vi "Station - Config File.vi"(6 "Action":enum16{"Write", "Read", "Read All", "Remove"}(ring), 8 "error in (no error)":errorcluster, 9 "Value":string[](array[string]), 10 "Key Name":string[](array[string]), 11 "Station Name":string) -> (0 "error out":errorcluster, 3 "Value Out":T1(array[cluster]))   [LabVIEW 2019]
uses:
  <vilib>/Utility/config.llb/Write Key (String).vi
  <vilib>/Utility/config.llb/Read Key (String).vi
  <vilib>/Utility/config.llb/NI_LVConfig.lvlib
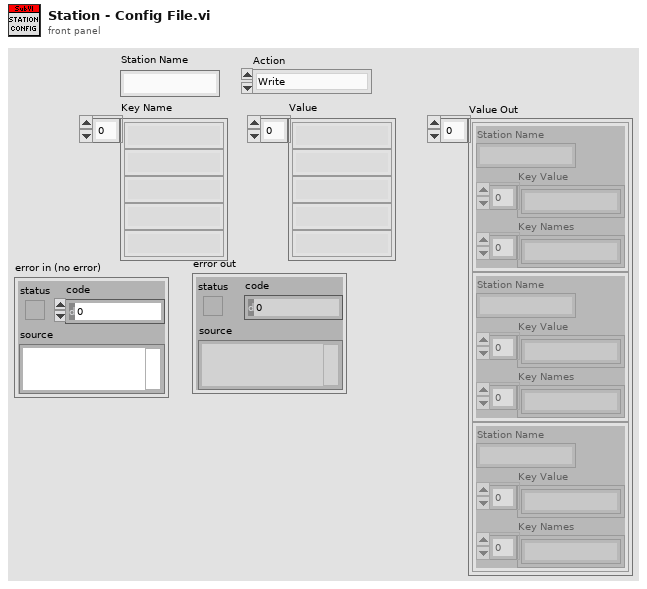
[diagram p1: front panel]
types:
  T1 = cluster{"Station Name":string, "Key Value":string[], "Key Names":string[]}[]
  T2 = typedef "NI_LVConfig.lvlib/Config Data RefNum.ctl" = refnum<k1>
  T3 = cluster{"Station Name":string, "Key Value":string[], "Key Names":string[]}
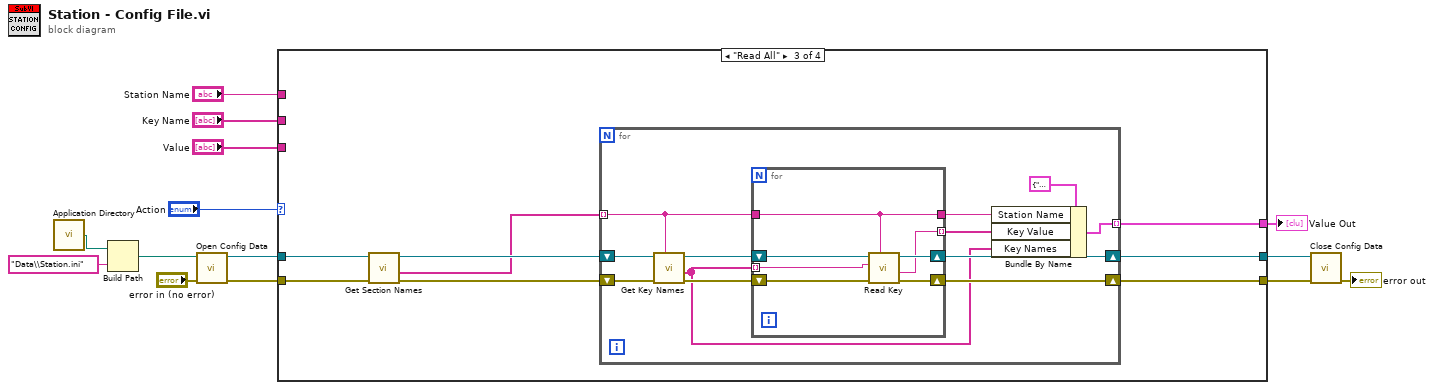
[diagram p0: block diagram]
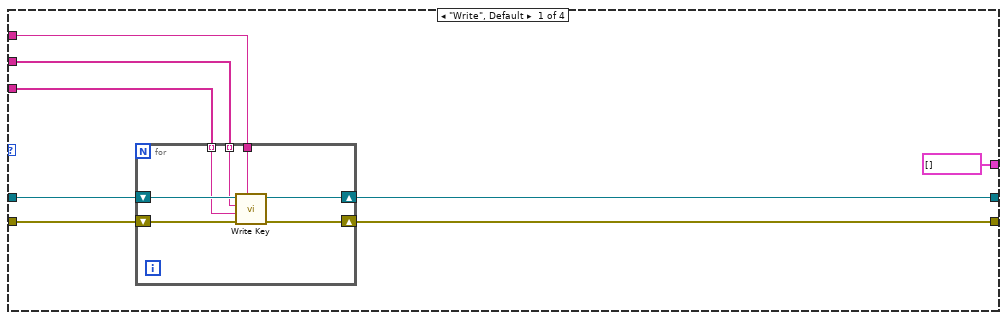
[diagram p2: hidden frame]
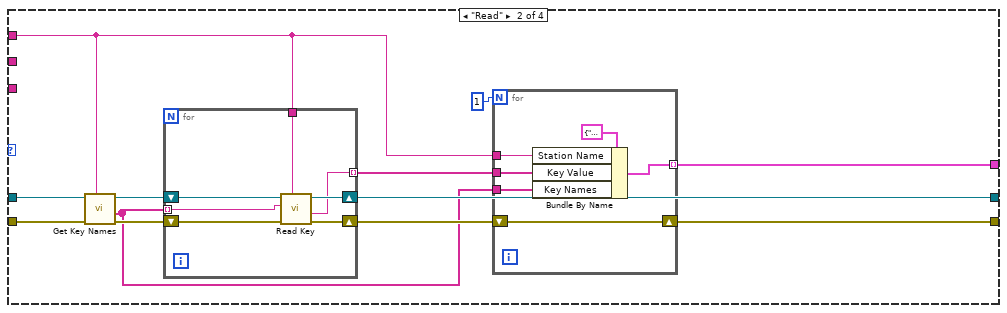
[diagram p3: hidden frame]
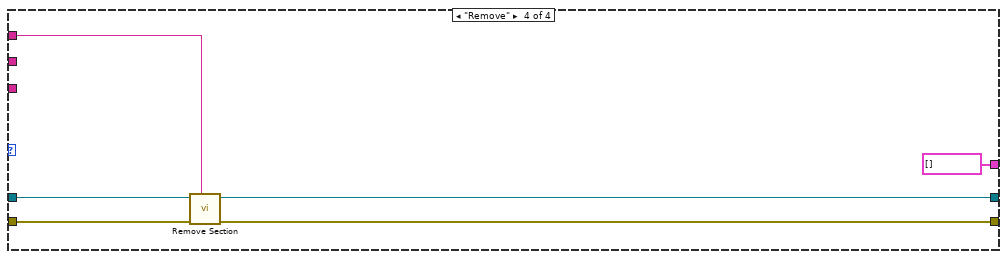
[diagram p4: hidden frame]
diagram:
  n1 = call <vilib>:"Application Directory.vi"() -> ("Application Directory"=w14:path)
  n2 = Build Path(base path=w14, name or relative path="Data\\Station.ini") -> (appended path=w1:path)
  n3 = call <vilib>:"Open Config Data.vi"("error in (no error)"="error in (no error)", "configuration file path"=w1) -> ("error out"=w12:errorcluster, "refnum"=w11:T2)  [unwired: 7 in, 1 out]
  n4 = case shown="\"Read All\"" "Action" {
    tunnel: w12 -> [w22 w34 w59 w85]
    tunnel: w11 -> [w21 w32 w58 w87]
    tunnel: [w20 w41 w61 w86] -> w10
    tunnel: [w19 w37 w62 w84] -> w9
    tunnel: "Value" -> [w18 _ _ _]
    tunnel: "Key Name" -> [w17 _ _ _]
    tunnel: "Station Name" -> [w16 w31 _ w83]
    tunnel: [T1 [] w39 w60 T1 []] -> w2
    frame "Write", Default {
      n5 = for {
        shift-right: [w26] -> w19
        shift-left: w22 -> [w29]
        shift-right: [w27] -> w20
        shift-left: w21 -> [w28]
        tunnel: w16 -> [w25]
        tunnel: w17 -> [w24] mode=indexing
        tunnel: w18 -> [w23] mode=indexing
        n6 = call-poly <vilib>:"Write Key.vi"("section"=w25, "error in (no error)"=w29, "value"=w23, "key"=w24, "refnum"=w28) -> ("error out"=w26:errorcluster, "refnum out"=w27:T2)  [unwired: 4 in, 1 out]
      }
    }
    frame "Read" {
      n7 = call <vilib>:"Get Key Names.vi"("section"=w31, "error in (no error)"=w34, "refnum"=w32) -> ("error out"=w35:errorcluster, "key names"=w30:string[], "refnum out"=w33:T2)  [unwired: 5 in, 1 out]
      n8 = for {
        tunnel: w31 -> [w50]
        shift-right: [w51] -> w41
        shift-left: w33 -> [w54]
        shift-right: [w52] -> w36
        shift-left: w35 -> [w53]
        tunnel: [w49] -> w40 mode=indexing
        tunnel: w30 -> [w48] mode=indexing
        n9 = call-poly <vilib>:"Read Key.vi"("section"=w50, "error in (no error)"=w53, "key"=w48, "refnum"=w54) -> ("error out"=w52:errorcluster, "value"=w49:string, "refnum out"=w51:T2)  [unwired: 4 in, 1 out]
      }
      n10 = for {
        N: 1 -> [_]
        tunnel: w31 -> [w47]
        tunnel: w40 -> [w46]
        tunnel: [w45] -> w39 mode=indexing
        shift-right: [w44] -> w37
        shift-left: w36 -> [w44]
        tunnel: w30 -> [w42]
        n11 = Bundle By Name(cluster=T3 {"Station Name"="", "Key Value"=[], "Key Names"=[]}, "Station Name"=w47, "Key Value"=w46, "Key Names"=w42) -> (w45:T3)
      }
    }
    frame "Read All" {
      n12 = call <vilib>:"Get Section Names.vi"("error in (no error)"=w59, "refnum"=w58) -> ("error out"=w57:errorcluster, "section names"=w55:string[], "refnum out"=w56:T2)  [unwired: 7 in]
      n13 = for {
        tunnel: [w64] -> w60 mode=indexing
        shift-right: [w74] -> w62
        shift-left: w57 -> [w72]
        shift-right: [w73] -> w61
        shift-left: w56 -> [w70]
        tunnel: w55 -> [w68] mode=indexing
        n14 = call <vilib>:"Get Key Names.vi"("section"=w68, "error in (no error)"=w72, "refnum"=w70) -> ("error out"=w71:errorcluster, "key names"=w63:string[], "refnum out"=w69:T2)  [unwired: 5 in, 1 out]
        n15 = for {
          shift-right: [w78] -> w73
          shift-left: w69 -> [w81]
          shift-right: [w79] -> w74
          shift-left: w71 -> [w80]
          tunnel: [w77] -> w65 mode=indexing
          tunnel: w63 -> [w76] mode=indexing
          tunnel: w68 -> [w75]
          tunnel: [w75] -> w66
          n16 = call-poly <vilib>:"Read Key.vi"("section"=w75, "error in (no error)"=w80, "key"=w76, "refnum"=w81) -> ("error out"=w79:errorcluster, "value"=w77:string, "refnum out"=w78:T2)  [unwired: 4 in, 1 out]
        }
        n17 = Bundle By Name(cluster=T3 {"Station Name"="", "Key Value"=[], "Key Names"=[]}, "Station Name"=w66, "Key Value"=w65, "Key Names"=w63) -> (w64:T3)
      }
    }
    frame "Remove" {
      n18 = call <vilib>:"Remove Section.vi"("section"=w83, "error in (no error)"=w85, "refnum"=w87) -> ("error out"=w84:errorcluster, "refnum out"=w86:T2)  [unwired: 6 in, 1 out]
    }
  }
  "Value Out" <- w2
  n19 = call <vilib>:"Close Config Data.vi"("error in (no error)"=w9, "refnum"=w10) -> ("error out"=→"error out":errorcluster)  [unwired: 8 in, 1 out]
